vi "AI generuj wektor konfiguracji kart.vi"(8 "error in (no error)":errorcluster, 11 "AI_param in":T2[](array[typedef]) {"Numer" min=1 max=8 step=1}) -> (0 "error out":errorcluster, 2 "HW konfig":T1[](array[typedef]))   [LabVIEW 2013]
doc: "Na podstawie ustawień kanałów analogowych (GUI)\nkonfiguruje ustawienia zakresu i aktywności filtru dla kart\nw przystawce"
uses:
  Kontrolki/GUI/AI_parametry.ctl
  Kontrolki/GUI/AI_wartosc.ctl
  Kontrolki/KartaDAQ/CONF AI HW config.ctl
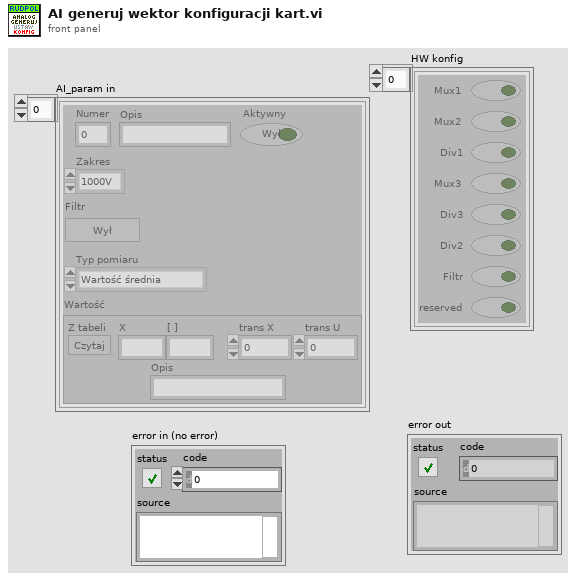
[diagram p1: front panel]
types:
  T1 = typedef "CONF AI HW config.ctl" = cluster{"Mux1":bool, "Mux2":bool, "Div1":bool, "Mux3":bool, "Div3":bool, "Div2":bool, "Filtr":bool, "reserved":bool}
  T2 = typedef "AI_parametry.ctl" = cluster{"Numer":u8, "Opis":string, "Zakres":enum16{"1000V", "300V", "30V", "3V", "0,3V"}, "Filtr":bool, "Typ pomiaru":enum16{"Wartość średnia", "Średnia wyprostowana", "Wartość skuteczna"}, "Aktywny":bool, "Wartość":T3}
  T3 = typedef "AI_wartosc.ctl" = cluster{"X":string, "[ ]":string, "trans X":dbl, "trans U":dbl, "Z tabeli":bool, "Opis":string}
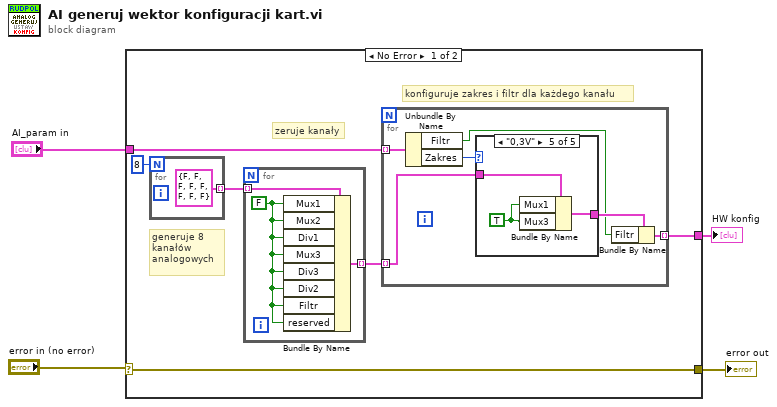
[diagram p0: block diagram]
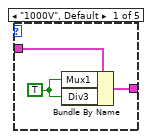
[diagram p2: hidden frame]
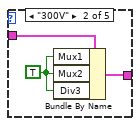
[diagram p3: hidden frame]
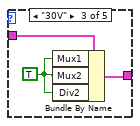
[diagram p4: hidden frame]
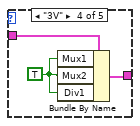
[diagram p5: hidden frame]
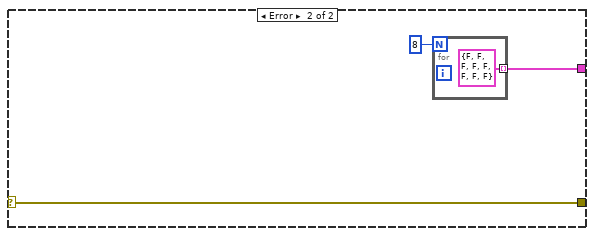
[diagram p6: hidden frame]
diagram:
  n1 = case shown="No Error" "error in (no error)" {
    selector: "error in (no error)" -> [w5 w38]
    tunnel: "AI_param in" -> [w7 _]
    tunnel: [w6 w37] -> w3
    tunnel: [w5 w38] -> w1
    frame No Error {
      # "konfiguruje zakres i filtr dla każdego kanału"
      # "zeruje kanały"
      # "generuje 8\nkanałów\nanalogowych"
      n2 = for {
        N: 8 -> [_]
        tunnel: [T1 {"Mux1"=FALSE, "Mux2"=FALSE, "Div1"=FALSE, "Mux3"=FALSE, "Div3"=FALSE, "Div2"=FALSE, "Filtr"=FALSE, "reserved"=FALSE} ("AI HW config")] -> w10 mode=indexing
      }
      n3 = for {
        tunnel: w10 -> [w14] mode=indexing
        tunnel: [w12] -> w8 mode=indexing
        w13 = FALSE ("Mux1")
        n4 = Bundle By Name(cluster=w14, "Mux1"=w13, "Mux2"=w13, "Div1"=w13, "Mux3"=w13, "Div3"=w13, "Div2"=w13, "Filtr"=w13, "reserved"=w13) -> (w12:T1)
      }
      n5 = for {
        tunnel: w7 -> [w20] mode=indexing
        tunnel: w8 -> [w18] mode=indexing
        tunnel: [w15] -> w6 mode=indexing
        n6 = Unbundle By Name(w20) -> ("Filtr"=w16:bool, "Zakres"=w19:enum16{"1000V", "300V", "30V", "3V", "0,3V"})
        n7 = case shown="\"0,3V\"" w19 {
          tunnel: w18 -> [w23 w26 w29 w31 w34]
          tunnel: [w21 w25 w27 w30 w33] -> w17
          frame "1000V", Default {
            w22 = TRUE ("Mux1")
            n8 = Bundle By Name(cluster=w23, "Mux1"=w22, "Div3"=w22) -> (w21:T1)
          }
          frame "300V" {
            w24 = TRUE ("Mux1")
            n9 = Bundle By Name(cluster=w26, "Mux1"=w24, "Mux2"=w24, "Div3"=w24) -> (w25:T1)
          }
          frame "30V" {
            w28 = TRUE ("Mux1")
            n10 = Bundle By Name(cluster=w29, "Mux1"=w28, "Mux2"=w28, "Div2"=w28) -> (w27:T1)
          }
          frame "3V" {
            w32 = TRUE ("Mux1")
            n11 = Bundle By Name(cluster=w31, "Mux1"=w32, "Mux2"=w32, "Div1"=w32) -> (w30:T1)
          }
          frame "0,3V" {
            w35 = TRUE ("Mux1")
            n12 = Bundle By Name(cluster=w34, "Mux1"=w35, "Mux3"=w35) -> (w33:T1)
          }
        }
        n13 = Bundle By Name(cluster=w17, "Filtr"=w16) -> (w15:T1)
      }
    }
    frame Error {
      n14 = for {
        N: 8 ("Numeric") -> [_]
        tunnel: [T1 {"Mux1"=FALSE, "Mux2"=FALSE, "Div1"=FALSE, "Mux3"=FALSE, "Div3"=FALSE, "Div2"=FALSE, "Filtr"=FALSE, "reserved"=FALSE} ("AI HW config")] -> w37 mode=indexing
      }
    }
  }
  "HW konfig" <- w3
  "error out" <- w1
